vi "Local Tracking Initialization.vi"(5 "Trajectory Cluster":T1, 6 "PID Cluster":T3={"L1 to L4 PID Cluster"={"L1 PID Gains"={"Kp"=0.005, "Kd"=0.5, "Ki"=0.0005}, "L2 PID Gains"={"Kp"=0.01, "Kd"=1.0, "Ki"=0.005}, "L3 PID Gains"={"Kp"=0.05, "Kd"=1.0, "Ki"=0.0005}, "L4 PID Gains"={"Kp"=0.1, "Kd"=0.1, "Ki"=0.0005}}, "Stage PID Cluster"={"Stage Z PID"={"Kp"=0.0005, "Kd"=0.001, "Ki"=0.0}, "Stage Y PID"={"Kp"=0.0003, "Kd"=0.01, "Ki"=0.0}, "Stage X PID"={"Kp"=0.0003, "Kd"=0.01, "Ki"=0.0}}, "OCT Z PID Gains"={"Kp"=0.0003, "Kd"=0.0001, "Ki"=0.01}}, 7 "Offset Home 2 RCM":dbl[](array[numeric])=[0.0, 0.0, 0.0, 0.0], 8 "error in":errorcluster, 10 "Prev Posit Cluster":T4={"Prev L1 to L4 Posit"=[0.0, 0.0, 0.0, 0.0], "Prev Stage Posit"=[6.0, 6.0, 6.0], "Prev OCT Z Posit"=0.0}, 11 "FPGA VI Reference In":refnum<k20>) -> (0 "error out":errorcluster, 2 "Last Posit Cluster":T2={"Last L1 to L4 Posit"=[0.0, 0.0, 0.0, 0.0], "Last Stage Posit"=[6.0, 6.0, 6.0], "Last OCT Z Posit"=0.0}, 3 "FPGA VI Reference Out":refnum<k20>)   [LabVIEW 2016]
uses:
  <vilib>/Platform/TimedLoop/XDataNode/timing_clust.ctl
  <vilib>/Platform/TimedLoop/XDataNode/nitl_modes.ctl
  <vilib>/Platform/TimedLoop/XDataNode/wakeup.ctl
  Global Variables.vi
  <vilib>/platform/TimedLoop/XDataNode/XDataNode.xnode
  <vilib>/Platform/TimedLoop/XDataNode/XDNodeRunTimeDep.lvlib
panel:
  out "In Servo Loop":bool
  out "Indexing Finished?":bool
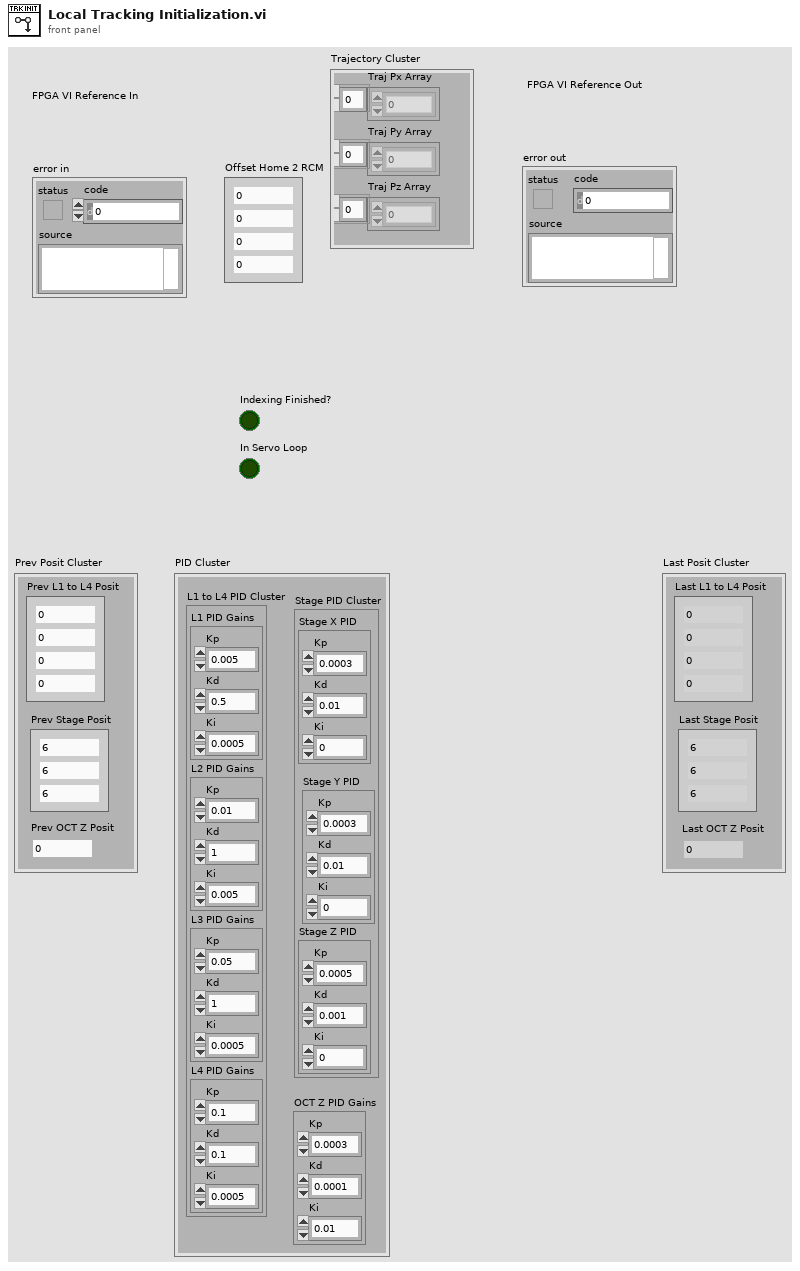
[diagram p1: front panel]
types:
  T1 = cluster{"Traj Px Array":dbl[], "Traj Py Array":dbl[], "Traj Pz Array":dbl[]}
  T2 = cluster{"Last L1 to L4 Posit":dbl[], "Last Stage Posit":dbl[], "Last OCT Z Posit":dbl}
  T3 = cluster{"L1 to L4 PID Cluster":cluster{"L1 PID Gains":cluster{"Kp":dbl, "Kd":dbl, "Ki":dbl}, "L2 PID Gains":cluster{"Kp":dbl, "Kd":dbl, "Ki":dbl}, "L3 PID Gains":cluster{"Kp":dbl, "Kd":dbl, "Ki":dbl}, "L4 PID Gains":cluster{"Kp":dbl, "Kd":dbl, "Ki":dbl}}, "Stage PID Cluster":cluster{"Stage Z PID":cluster{"Kp":dbl, "Kd":dbl, "Ki":dbl}, "Stage Y PID":cluster{"Kp":dbl, "Kd":dbl, "Ki":dbl}, "Stage X PID":cluster{"Kp":dbl, "Kd":dbl, "Ki":dbl}}, "OCT Z PID Gains":cluster{"Kp":dbl, "Kd":dbl, "Ki":dbl}}
  T4 = cluster{"Prev L1 to L4 Posit":dbl[], "Prev Stage Posit":dbl[], "Prev OCT Z Posit":dbl}
  T5 = typedef "XDNodeRunTimeDep.lvlib/timing_clust.ctl" = cluster{"Expected End [f-1]":u64, "Actual End [f-1]":u64, "Finished Late? [f-1]":bool, "Expected End [i-1]":u64, "Actual End [i-1]":u64, "Finished Late? [i-1]":bool, "Expected Start [i]":u64, "Actual Start [i]":u64, "Expected Start [f]":u64, "Actual Start [f]":u64, "Source Name":string, "Structure Name":string, "Period":i64, "Deadline":i64, "Offset":i64, "Start":i64, "Priority":i32, "Timeout":i32, "Mode":T6, "Wakeup Reason":T7, "Error":errorcluster, "Source Type":string, "Secondary Source Type":string, "Global End Time":u64, "Global Start Time":u64, "Frame Duration":u64, "Iteration Duration":u64, "Assigned CPU":i32, "I/O Scan Engine Mode":u32}
  T6 = typedef "XDNodeRunTimeDep.lvlib/nitl_modes.ctl" = enum32{"No Change", "Process missed periods, maintain original phase", "Discard missed periods, maintain original phase", "Process missed periods, ignore original phase", "Discard missed periods, ignore original phase"}
  T7 = typedef "XDNodeRunTimeDep.lvlib/wakeup.ctl" = enum32{"Normal", "Aborted", "Asynchronous wakeup", "Timing source error", "Timed loop error", "Timeout"}
  T8 = cluster{"L1 PID Gains":cluster{"Kp":dbl, "Kd":dbl, "Ki":dbl}, "L2 PID Gains":cluster{"Kp":dbl, "Kd":dbl, "Ki":dbl}, "L3 PID Gains":cluster{"Kp":dbl, "Kd":dbl, "Ki":dbl}, "L4 PID Gains":cluster{"Kp":dbl, "Kd":dbl, "Ki":dbl}}
  T9 = cluster{"Stage Z PID":cluster{"Kp":dbl, "Kd":dbl, "Ki":dbl}, "Stage Y PID":cluster{"Kp":dbl, "Kd":dbl, "Ki":dbl}, "Stage X PID":cluster{"Kp":dbl, "Kd":dbl, "Ki":dbl}}
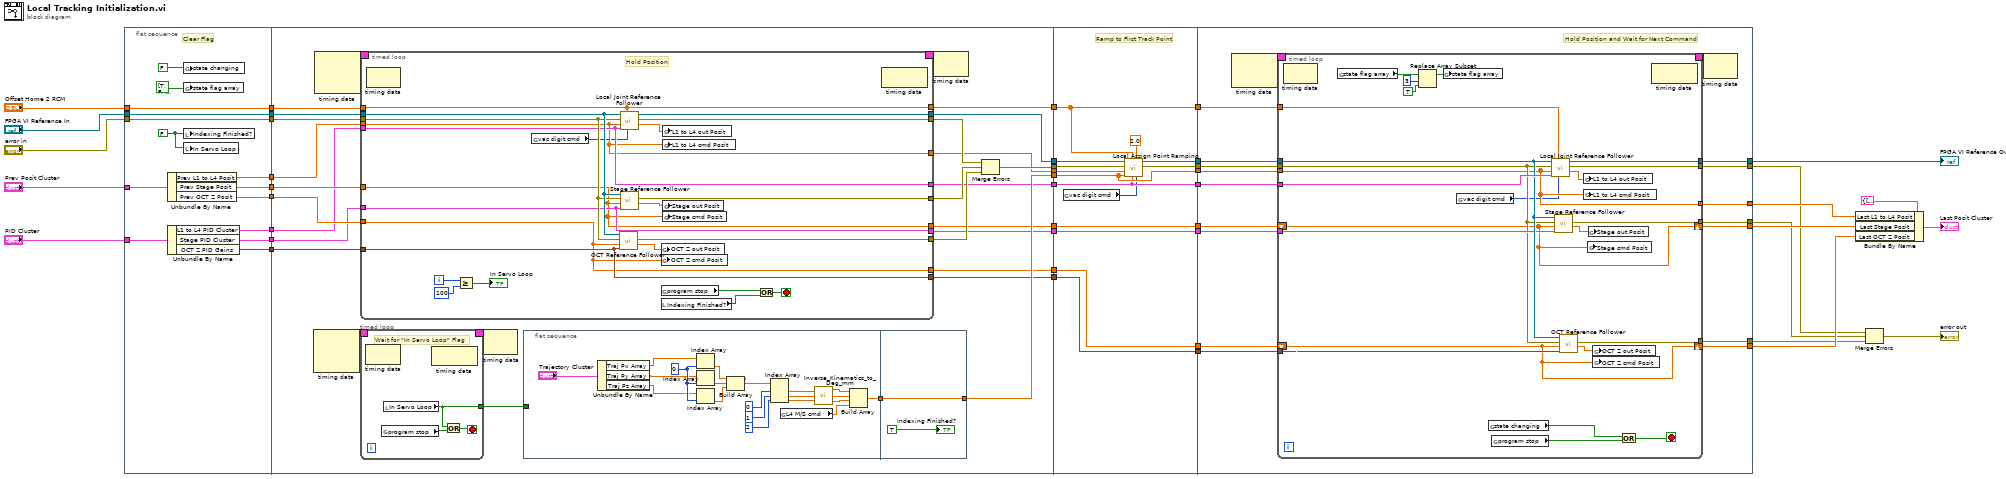
[diagram p0: block diagram]
diagram:
  n1 = flat-sequence {
    tunnel: [w55] -> w21
    tunnel: "FPGA VI Reference In" -> [w55]
    tunnel: "error in" -> [w54]
    tunnel: [w54] -> w19
    tunnel: [w49] -> w17
    tunnel: "PID Cluster" -> [w48]
    tunnel: "Offset Home 2 RCM" -> [w53]
    tunnel: [w53] -> w15
    tunnel: "Prev Posit Cluster" -> [w52]
    tunnel: [w51] -> w12
    tunnel: [w50] -> w10
    tunnel: [w47] -> w8
    tunnel: [w46] -> w7
    tunnel: [w45] -> w6
    tunnel: w21 -> [w82]
    tunnel: [w76] -> w20
    tunnel: w19 -> [w81]
    tunnel: [w72] -> w18
    tunnel: w17 -> [w80]
    tunnel: [w71] -> w16
    tunnel: w15 -> [w83]
    tunnel: [w77] -> w14
    tunnel: [w70] -> w13
    tunnel: w12 -> [w79]
    tunnel: [w68] -> w11
    tunnel: w10 -> [w78]
    tunnel: [w69] -> w9
    tunnel: w8 -> [w67]
    tunnel: w7 -> [w66]
    tunnel: w6 -> [w65]
    tunnel: [w64] -> w5
    tunnel: [w63] -> w3
    tunnel: [w62] -> w1
    tunnel: w20 -> [w155]
    tunnel: w18 -> [w154]
    tunnel: w16 -> [w152]
    tunnel: w14 -> [w149]
    tunnel: w13 -> [w148]
    tunnel: [w151] -> w41
    tunnel: [w148] -> w40
    tunnel: [w150] -> w39
    tunnel: [w149] -> w38
    tunnel: [w145] -> w35
    tunnel: [w143] -> w34
    tunnel: w11 -> [w147]
    tunnel: [w147] -> w22
    tunnel: w9 -> [w144]
    tunnel: w5 -> [w146]
    tunnel: [w146] -> w4
    tunnel: w3 -> [w145]
    tunnel: [w144] -> w2
    tunnel: w1 -> [w143]
    tunnel: [w168] -> w30
    tunnel: [w167] -> w25
    tunnel: w41 -> [w170]
    tunnel: w40 -> [w157]
    tunnel: w39 -> [w171]
    tunnel: w38 -> [w158]
    tunnel: [w166] -> w36
    tunnel: [w165] -> w37
    tunnel: w35 -> [w164]
    tunnel: w34 -> [w163]
    tunnel: [w162] -> w31
    tunnel: [w161] -> w24
    tunnel: [w160] -> w23
    tunnel: w22 -> [w159]
    tunnel: w4 -> [w169]
    tunnel: w2 -> [w156]
    frame #0 {
      w44 = FALSE ("Indexing Finished?")
      # "Clear Flag"
      n2 = Unbundle By Name(w52) -> ("Prev L1 to L4 Posit"=w49:dbl[], "Prev Stage Posit"=w51:dbl[], "Prev OCT Z Posit"=w50:dbl)
      n3 = Unbundle By Name(w48) -> ("L1 to L4 PID Cluster"=w47:T8, "Stage PID Cluster"=w46:T9, "OCT Z PID Gains"=w45:cluster{"Kp":dbl, "Kd":dbl, "Ki":dbl})
      n4 = global write "Global Variables.vi" "state changing"(FALSE ("state changing")) -> ()
      n5 = global write "Global Variables.vi" "state flag array"(bool[] [TRUE, FALSE, FALSE, FALSE, FALSE, FALSE, FALSE, FALSE, FALSE] ("state flag array")) -> ()
      n6 = local write "Indexing Finished?"(w44) -> ()
      n7 = local write "In Servo Loop"(w44) -> ()
    }
    frame #1 {
      n8 = node-c288() -> (w61:T5)  [unwired: 3 in]
      n9 = node-c288() -> (w85:T5)  [unwired: 3 in]
      n10 = timed-loop {
        timing: w61 -> [_]
        timing-out: [_] -> w60
        tunnel: [w108] -> w59
        stop <- w110 stop-if-true
        # "Wait for \"In Servo Loop\" Flag"
        n11 = node-c288() -> ()  [unwired: 1 in, 1 out]
        n12 = global read "Global Variables.vi" "program stop"() -> (w109:bool)
        n13 = local read "In Servo Loop"() -> (w108:bool)
        n14 = node-c288() -> ()  [unwired: 1 in, 1 out]
        n15 = Or(x=w108, y=w109) -> (x .or. y?=w110:bool)
      }
      n16 = timed-loop {
        timing: w85 -> [_]
        timing-out: [_] -> w84
        tunnel: w83 -> [w135]
        tunnel: w82 -> [w137]
        tunnel: w81 -> [w136]
        tunnel: w80 -> [w118]
        tunnel: w79 -> [w117]
        tunnel: w78 -> [w116]
        tunnel: [w135] -> w77
        tunnel: [w134] -> w76
        tunnel: [w133] -> w75
        tunnel: [w132] -> w74
        tunnel: [w131] -> w73
        tunnel: [w118] -> w71
        tunnel: [w117] -> w68
        tunnel: [w116] -> w69
        tunnel: w67 -> [w124]
        tunnel: w66 -> [w123]
        tunnel: w65 -> [w122]
        tunnel: [w124] -> w64
        tunnel: [w123] -> w63
        tunnel: [w122] -> w62
        i -> [w121]
        stop <- w126 stop-if-true
        # "Hold Position"
        n17 = node-c288() -> ()  [unwired: 1 in, 1 out]
        n18 = Greater Or Equal?(x=w121, y=100) -> (x >= y?=→"In Servo Loop":bool)
        n19 = global read "Global Variables.vi" "vac digit cmd"() -> (w115:i8)
        n20 = call "OCT Reference Follower.vi"("OCT Z PID Gains"=w122, "OCT  Z cmd Posit [mm]"=w116, "error in"=w136, "FPGA VI Reference In"=w137) -> ("OCT  Z out Posit [mm]"=w128:dbl, "error out"=w131:errorcluster)  [unwired: 5 in, 1 out]
        n21 = call "Local Joint Reference Follower.vi"("Digital Cmd [0-78]"=w115, "Offset Home2RCM [deg/mm]"=w135, "PID Ctrl Cluster"=w124, "Ref Array [deg/mm]"=w118, "error in"=w136, "FPGA VI Reference In"=w137) -> ("Output Posit Array [deg/mm]"=w130:dbl[], "error out"=w133:errorcluster, "FPGA VI Reference Out"=w134:refnum<k20>)  [unwired: 3 in]
        n22 = call "Stage Reference Follower.vi"("Stage PID Cluster"=w123, "Stage cmd Posit [mm]"=w117, "error in"=w136, "FPGA VI Reference In"=w137) -> ("Stage out Posit [mm]"=w129:dbl[], "error out"=w132:errorcluster)  [unwired: 5 in, 1 out]
        n23 = global write "Global Variables.vi" "OCT Z out Posit"(w128) -> ()
        n24 = global write "Global Variables.vi" "OCT Z cmd Posit"(w116) -> ()
        n25 = global read "Global Variables.vi" "program stop"() -> (w127:bool)
        n26 = local read "Indexing Finished?"() -> (w125:bool)
        n27 = global write "Global Variables.vi" "L1 to L4 out Posit"(w130) -> ()
        n28 = global write "Global Variables.vi" "L1 to L4 cmd Posit"(w118) -> ()
        n29 = global write "Global Variables.vi" "Stage out Posit"(w129) -> ()
        n30 = global write "Global Variables.vi" "Stage cmd Posit"(w117) -> ()
        n31 = Or(x=w127, y=w125) -> (x .or. y?=w126:bool)
        n32 = node-c288() -> ()  [unwired: 1 in, 1 out]
      }
      n33 = node-c288(w60) -> ()  [unwired: 1 out]
      n34 = flat-sequence {
        tunnel: w59 -> [_]
        tunnel: [w87] -> w58
        tunnel: [w106] -> w70
        tunnel: w58 -> [w106]
        frame #0 {
          w92 = 0 ("index")
          n35 = Unbundle By Name("Trajectory Cluster") -> ("Traj Px Array"=w88:dbl[], "Traj Py Array"=w90:dbl[], "Traj Pz Array"=w89:dbl[])
          n36 = Index Array(array=w88, index=w92) -> (element=w104:dbl)
          n37 = Index Array(array=w90, index=w92) -> (element=w103:dbl)
          n38 = Index Array(array=w89, index=w92) -> (element=w102:dbl)
          n39 = Build Array(w104, w103, w102) -> (w91:dbl[])
          n40 = Index Array(array=w91, index #1=0 ("index"), index #2=1 ("index"), index #3=2 ("index")) -> (element #1=w97:dbl, element #2=w95:dbl, element #3=w96:dbl)
          n41 = global read "Global Variables.vi" "L4 M/S cmd"() -> (w86:dbl)
          n42 = call "Inverse_Kinematics_to_Deg_mm.vi"("pz"=w96, "py"=w95, "px"=w97) -> ("L3 [mm]"=w100:dbl, "L2 [deg]"=w99:dbl, "L1 [deg]"=w98:dbl)
          n43 = Build Array(w98, w99, w100, w86) -> (w87:dbl[])
        }
        frame #1 {
          "Indexing Finished?" <- TRUE ("Indexing Finished?")
        }
      }
      n44 = node-c288(w84) -> ()  [unwired: 1 out]
      n45 = Merge Errors(w75, w74, w73) -> (w72:errorcluster)
    }
    frame #2 {
      # "Ramp to First Track Point"
      n46 = global read "Global Variables.vi" "vac digit cmd"() -> (w142:i8)
      n47 = call "Local Assign Point Ramping.vi"("Vac Digital Cmd"=w142, "Ramp Time [sec]"=2.0, "L1 to L4 PID Cluster"=w146, "Offset Home2RCM"=w149, "Destination Posit Array [mm]"=w148, "Previous Posit Array"=w152, "error in"=w154, "FPGA VI Reference In"=w155) -> ("error out"=w151:errorcluster, "FPGA VI Reference Out"=w150:refnum<k20>)  [unwired: 1 in, 1 out]
    }
    frame #3 {
      # "Hold Position and Wait for Next Command"
      n48 = node-c288() -> (w173:T5)  [unwired: 2 in]
      n49 = timed-loop {
        timing: w173 -> [_]
        timing-out: [_] -> w172
        tunnel: w171 -> [w187]
        tunnel: w170 -> [w180]
        tunnel: w158 -> [w192]
        tunnel: w157 -> [w177]
        tunnel: w169 -> [w191]
        tunnel: [w190] -> w168
        tunnel: [w189] -> w167
        tunnel: [w177] -> w166
        tunnel: w164 -> [w184]
        tunnel: w163 -> [w183]
        tunnel: [w179] -> w161
        tunnel: [w178] -> w160
        shift-right: [w176] -> w165
        shift-left: w159 -> [w176]
        shift-right: [w175] -> w162
        shift-left: w156 -> [w175]
        stop <- w181 stop-if-true
        # "Hold Position if not Engaged"
        n50 = node-c288() -> ()  [unwired: 1 in, 1 out]
        n51 = global read "Global Variables.vi" "state flag array"() -> (w196:bool[])
        n52 = Replace Array Subset(array=w196, new element=TRUE ("new element/subarray"), index=3) -> (w195:bool[])
        n53 = global write "Global Variables.vi" "state flag array"(w195) -> ()
        n54 = global read "Global Variables.vi" "vac digit cmd"() -> (w174:i8)
        n55 = global read "Global Variables.vi" "state changing"() -> (w197:bool)
        n56 = global read "Global Variables.vi" "program stop"() -> (w186:bool)
        n57 = call "Local Joint Reference Follower.vi"("Digital Cmd [0-78]"=w174, "Offset Home2RCM [deg/mm]"=w192, "PID Ctrl Cluster"=w191, "Ref Array [deg/mm]"=w177, "error in"=w180, "FPGA VI Reference In"=w187) -> ("Output Posit Array [deg/mm]"=w185:dbl[], "error out"=w189:errorcluster, "FPGA VI Reference Out"=w190:refnum<k20>)  [unwired: 3 in]
        n58 = call "Stage Reference Follower.vi"("Stage PID Cluster"=w184, "Stage cmd Posit [mm]"=w176, "error in"=w180, "FPGA VI Reference In"=w187) -> ("Stage out Posit [mm]"=w188:dbl[], "error out"=w179:errorcluster)  [unwired: 5 in, 1 out]
        n59 = call "OCT Reference Follower.vi"("OCT Z PID Gains"=w183, "OCT  Z cmd Posit [mm]"=w175, "error in"=w180, "FPGA VI Reference In"=w187) -> ("OCT  Z out Posit [mm]"=w182:dbl, "error out"=w178:errorcluster)  [unwired: 5 in, 1 out]
        n60 = global write "Global Variables.vi" "L1 to L4 out Posit"(w185) -> ()
        n61 = global write "Global Variables.vi" "L1 to L4 cmd Posit"(w177) -> ()
        n62 = global write "Global Variables.vi" "Stage cmd Posit"(w176) -> ()
        n63 = global write "Global Variables.vi" "Stage out Posit"(w188) -> ()
        n64 = global write "Global Variables.vi" "OCT Z out Posit"(w182) -> ()
        n65 = global write "Global Variables.vi" "OCT Z cmd Posit"(w175) -> ()
        n66 = Or(x=w197, y=w186) -> (x .or. y?=w181:bool)
        n67 = node-c288() -> ()  [unwired: 1 in, 1 out]
      }
      n68 = node-c288(w172) -> ()  [unwired: 1 out]
    }
  }
  n69 = Bundle By Name(cluster=T2 {"Last L1 to L4 Posit"=[0.0, 0.0, 0.0, 0.0], "Last Stage Posit"=[6.0, 6.0, 6.0], "Last OCT Z Posit"=0.0} ("Last Posit Cluster 2"), "Last L1 to L4 Posit"=w36, "Last Stage Posit"=w37, "Last OCT Z Posit"=w31) -> (→"Last Posit Cluster":T2)
  n70 = Merge Errors(w25, w24, w23) -> (→"error out":errorcluster)
  "FPGA VI Reference Out" <- w30
